vi "__init__.vi"(8 "error in (no error)":errorcluster, 11 "self in":refnum<class "Identifier.lvclass">) -> (0 "error out":errorcluster, 3 "self out":refnum<class "Identifier.lvclass">)   [LabVIEW 2020, in "mlir.lvlib" / "Identifier.lvclass"]
uses:
  Identifier.lvclass
  Identifier.lvclass/Identifier.ctl
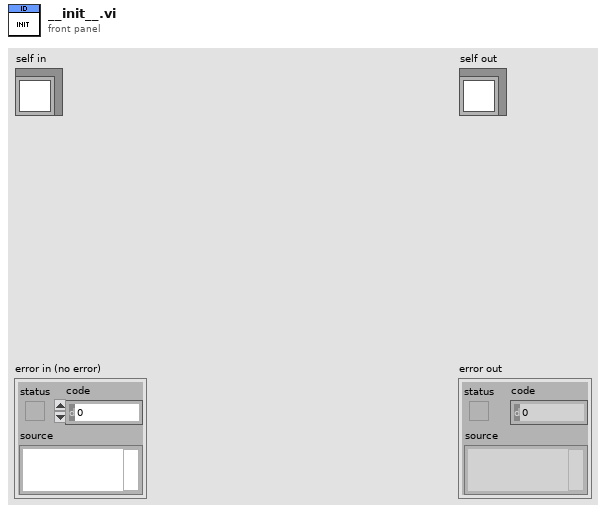
[diagram p1: front panel]
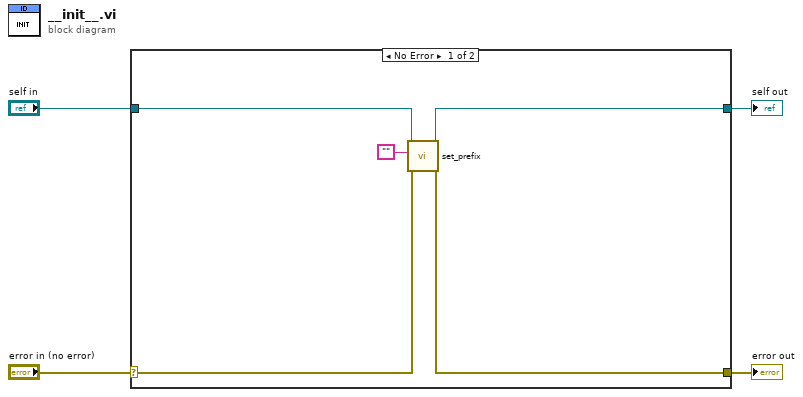
[diagram p0: block diagram]
diagram:
  n1 = case shown="No Error" "error in (no error)" {
    selector: "error in (no error)" -> [w7 w11]
    tunnel: [w6 w11] -> w3
    tunnel: [w9 w10] -> w1
    tunnel: "self in" -> [w8 w10]
    frame No Error {
      n2 = call-dynamic "set_prefix.vi"("error in (no error)"=w7, "_prefix_"="", "Identifier in"=w8) -> ("error out"=w6:errorcluster, "Identifier out"=w9:refnum<class "Identifier.lvclass">)  [unwired: 7 in]
    }
    frame Error {
    }
  }
  "error out" <- w3
  "self out" <- w1
